vi "GV_TagProperties_GetOne.vi"(1 "TAG":string, 2 "TAGproperties":T3 {"TAGprop"."TagFunc" format="%08x"; "TAGprop"."RangeL" format="%.2f"; "TAGprop"."RangeH" format="%.2f"}) -> (6 "TAGproperty":T1 {"TAGprop"."TagFunc" format="%08x"; "TAGprop"."RangeL" format="%.2f"; "TAGprop"."RangeH" format="%.2f"})   [LabVIEW 2020, in "Sgraph_lib_V1.lvlib" / "Gviewer.lvclass"]
doc: "Andre Koelewijn, 3 mar 2022 : get one tag properties from the tag properties array by TAG name"
uses:
  Gviewer.lvclass
  DBAL/controls/DBAL_TAGprops.ctl
  DBAL/controls/DBAL_TAGpropEdit.ctl
  Common/controls/typedef_com_TagProp.ctl
  Builds/Sgraph_lib_V1.lvlib
  DBAL/DBAL.lvclass
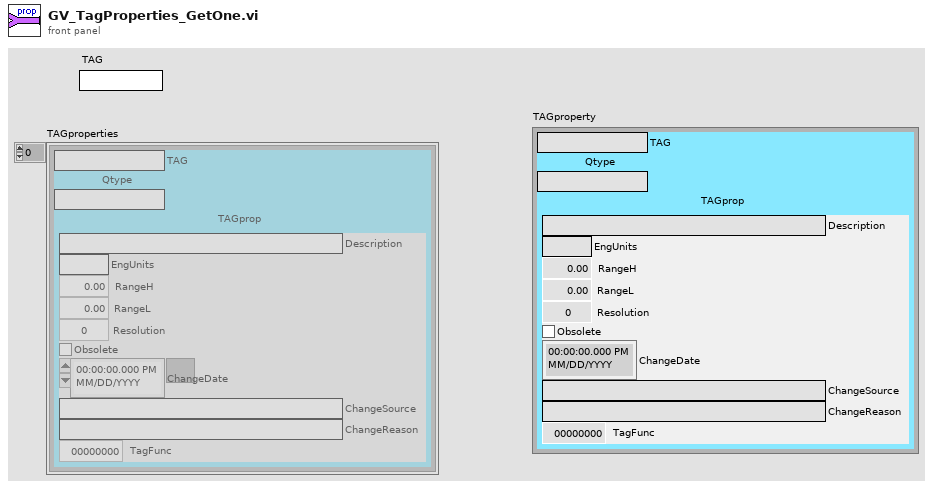
[diagram p1: front panel]
types:
  T1 = typedef "Sgraph_lib_V1.lvlib/DBAL.lvclass/DBAL_TAGpropEdit.ctl" = cluster{"TAG":string, "Qtype":string, "TAGprop":T2}
  T2 = typedef "Sgraph_lib_V1.lvlib/typedef_com_TagProp.ctl" = cluster{"Description":string, "EngUnits":string, "RangeH":dbl, "RangeL":dbl, "Resolution":i32, "Obsolete":bool, "ChangeDate":timestamp, "ChangeSource":string, "ChangeReason":string, "TagFunc":u32}
  T3 = typedef "Sgraph_lib_V1.lvlib/DBAL.lvclass/DBAL_TAGprops.ctl" = T1[]
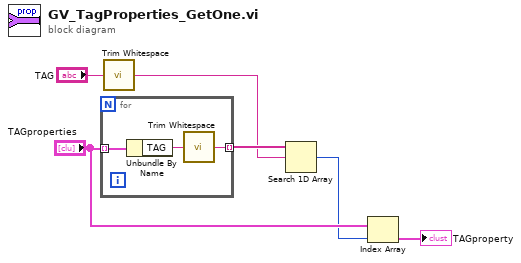
[diagram p0: block diagram]
diagram:
  n1 = for {
    tunnel: "TAGproperties" -> [w9] mode=indexing
    tunnel: [w7] -> w5 mode=indexing
    n2 = Unbundle By Name(w9) -> ("TAG"=w8:string)
    n3 = call <vilib>:"Trim Whitespace.vi"("string"=w8) -> ("trimmed string"=w7:string)  [unwired: 1 in]
  }
  n4 = call <vilib>:"Trim Whitespace.vi"("string"="TAG") -> ("trimmed string"=w4:string)  [unwired: 1 in]
  n5 = Search 1D Array(1D array=w5, element=w4) -> (index of element=w2:i32)  [unwired: 1 in]
  n6 = Index Array(array="TAGproperties", index=w2) -> (element=→"TAGproperty":T1)
